vi "Run Measurement.vi"(4 "Iterations":i32=1, 6 "Show FP?":bool=TRUE, 7 "Continuous Run":bool, 8 "error in (no error)":errorcluster, 9 "Device Names":string[](array[string]), 10 "Measurement Name":string, 11 "Self Enqueuer In":refnum<class "Message Enqueuer.lvclass">) -> (0 "error out":errorcluster, 2 "Measurement Results":refnum<class "Results.lvclass">, 3 "Self Enqueuer Out":refnum<class "Message Enqueuer.lvclass">)   [LabVIEW 2026, in "Controller API.lvlib" / "Controller API.lvclass"]
uses:
  Controller API.lvclass
  Controller API.lvclass/Controller API.ctl
  Messages/Launch Measurement Msg/Launch Measurement and Wait for Result.lvclass
  C:/Users/E2013170/Documents/GitHub/Measurement-Utility-Reference/components/MAL-Framework/user.lib/Common Components/Controller/Messages/Launch Measurements Message/Launch Measurements Message.lvclass
  C:/Program Files/National Instruments/LabVIEW 2026/vi.lib/ActorFramework/Message/Message.lvclass
  C:/Users/E2013170/Documents/GitHub/Measurement-Utility-Reference/components/MAL-Framework-API/Messages/Launch Measurement Msg/Launch Measurement and Wait for Result.lvclass
  MAL-Framework/user.lib/Common Components/Results/Results.lvclass
  MAL-Framework/user.lib/Common Components/Controller/Messages/Launch Measurements Message/Launch Measurements Message.lvclass
  <vilib>/ActorFramework/Message Enqueuer/Message Enqueuer.lvclass
  Error Result/Error Report.lvclass
panel:
  out "error out 2":errorcluster
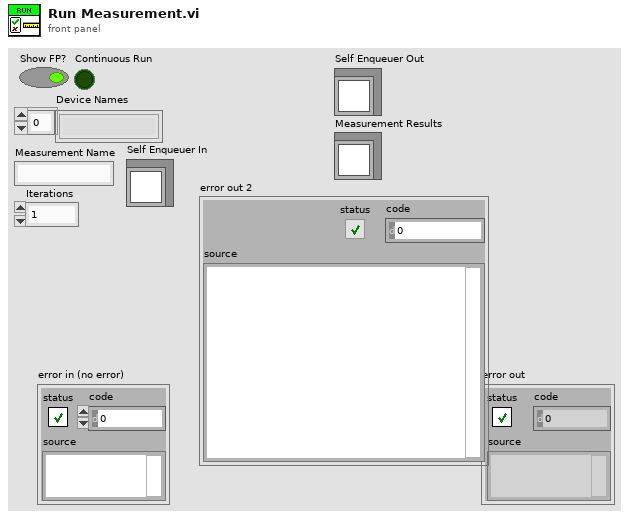
[diagram p1: front panel]
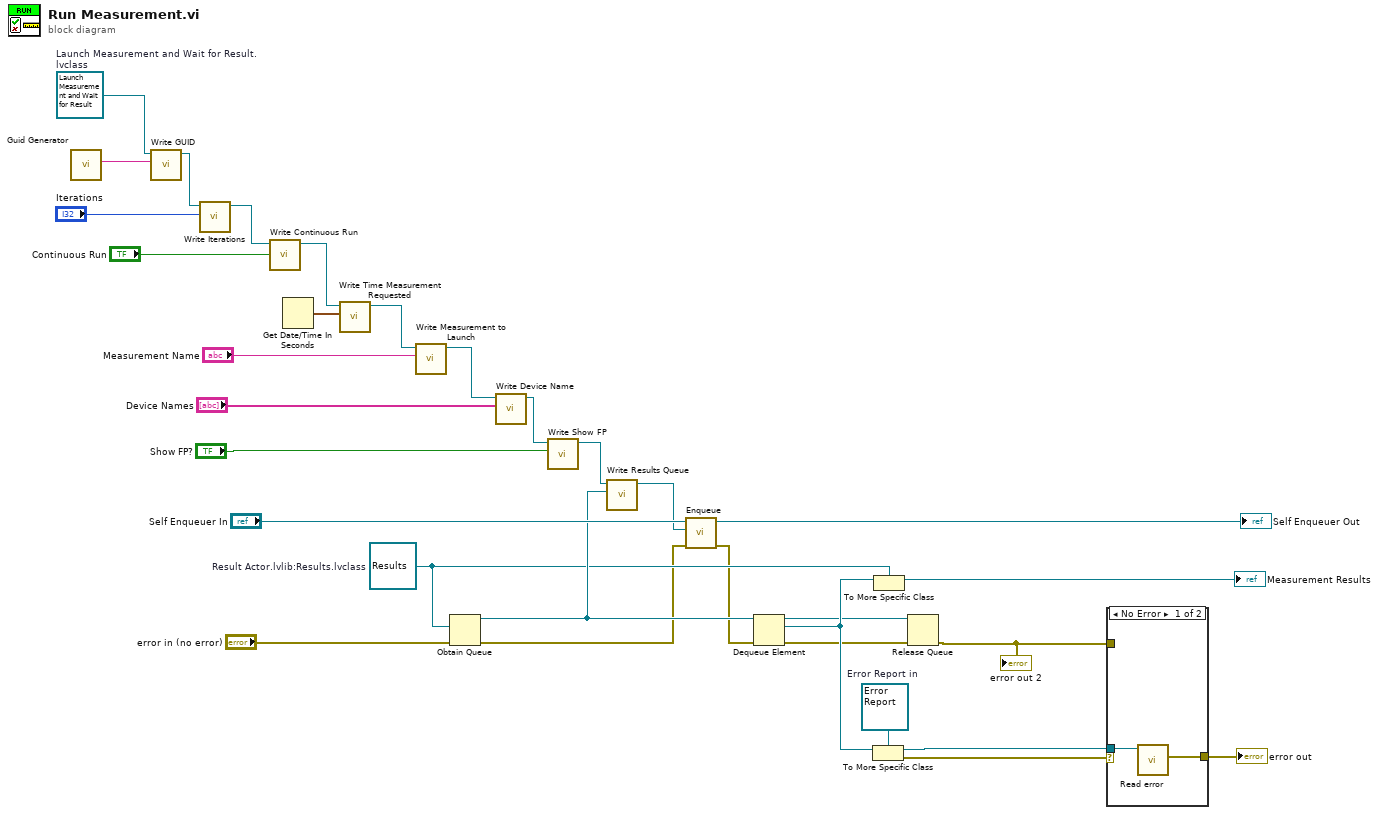
[diagram p0: block diagram]
diagram:
  w14 = refnum<class "Error Report.lvclass"> refnum  # Error Report in
  w6 = refnum<class "Launch Measurement and Wait for Result.lvclass"> refnum  # Launch Measurement and Wait for Result.lvclass
  w10 = refnum<class "Results.lvclass"> refnum  # Result Actor.lvlib:Results.lvclass
  n1 = call "Guid Generator.vi"() -> ("GUID"=w19:string)  [unwired: 10 in, 1 out]
  n2 = call "Write GUID.vi"("GUID"=w19, "Launch Measurements Message in"=w6) -> ("Launch Measurements Message out"=w3:refnum<class "Launch Measurement and Wait for Result.lvclass">)  [unwired: 8 in, 1 out]
  n3 = call "Write Iterations.vi"("Iterations"="Iterations", "Launch Measurements Message in"=w3) -> ("Launch Measurements Message out"=w2:refnum<class "Launch Measurement and Wait for Result.lvclass">)  [unwired: 8 in, 1 out]
  n4 = call "Write Continuous Run.vi"("Continuous Run"="Continuous Run", "Launch Measurements Message in"=w2) -> ("Launch Measurements Message out"=w5:refnum<class "Launch Measurement and Wait for Result.lvclass">)  [unwired: 8 in, 1 out]
  n5 = Get Date/Time In Seconds() -> (seconds since 1Jan1904=w20:timestamp)
  n6 = call "Write Time Measurement Requested.vi"("Time Measurement Requested"=w20, "Launch Measurements Message in"=w5) -> ("Launch Measurements Message out"=w21:refnum<class "Launch Measurement and Wait for Result.lvclass">)  [unwired: 8 in, 1 out]
  n7 = call "Write Measurement to Launch.vi"("Measurement Name"="Measurement Name", "Launch Measurements Message in"=w21) -> ("Launch Measurements Message out"=w30:refnum<class "Launch Measurement and Wait for Result.lvclass">)  [unwired: 8 in, 1 out]
  n8 = Obtain Queue(element data type=w10, error in (no error)="error in (no error)") -> (queue out=w27:refnum<queue>, error out=w9:errorcluster)  [unwired: 3 in, 1 out]
  n9 = call "Write Device Name.vi"("Device Names"="Device Names", "Launch Measurements Message in"=w30) -> ("Launch Measurements Message out"=w29:refnum<class "Launch Measurement and Wait for Result.lvclass">)  [unwired: 8 in, 1 out]
  n10 = call "Write Show FP.vi"("Show FP?"="Show FP?", "Launch Measurements Message in"=w29) -> ("Launch Measurements Message out"=w28:refnum<class "Launch Measurement and Wait for Result.lvclass">)  [unwired: 8 in, 1 out]
  n11 = call "Write Results Queue.vi"("Results Queue"=w27, "Launch Measurement and Wait for Result in"=w28) -> ("Launch Measurement and Wait for Result out"=w23:refnum<class "Launch Measurement and Wait for Result.lvclass">)  [unwired: 8 in, 1 out]
  n12 = call <vilib>:"Enqueue.vi"("error in (no error)"=w9, "Message"=w23, "Message Enqueuer in"="Self Enqueuer In") -> ("error out"=w8:errorcluster, "Message Enqueuer out"=→"Self Enqueuer Out":refnum<class "Message Enqueuer.lvclass">)  [unwired: 7 in]
  n13 = Dequeue Element(queue=w27, error in (no error)=w8) -> (queue out=w12:refnum<queue>, element=w17:refnum<class "Results.lvclass">, error out=w11:errorcluster)  [unwired: 1 in, 1 out]
  n14 = To More Specific Class(target class=w14, reference=w17) -> (specific class reference=w13:refnum<class "Error Report.lvclass">, error out=w16:errorcluster)  [unwired: 1 in]
  n15 = To More Specific Class(target class=w10, reference=w17) -> (specific class reference=→"Measurement Results":refnum<class "Results.lvclass">)  [unwired: 1 in, 1 out]
  n16 = Release Queue(queue=w12, error in (no error)=w11) -> (error out=w7:errorcluster)  [unwired: 1 in, 2 out]
  "error out 2" <- w7
  n17 = case shown="No Error" w16 {
    tunnel: w13 -> [w34 _]
    tunnel: [w33 w35] -> w15
    tunnel: w7 -> [_ w35]
    frame No Error {
      n18 = call "Read error.vi"("Error Report in"=w34) -> ("error"=w33:errorcluster)  [unwired: 8 in, 2 out]
    }
    frame Error {
    }
  }
  "error out" <- w15
